vi "Flush Registry.vi"(8 "error in":errorcluster) -> (0 "error out":errorcluster)   [LabVIEW 2019, in "Identifier.lvclass"]
uses:
  Identifier.lvclass
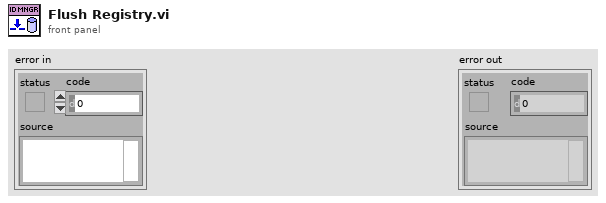
[diagram p1: front panel]
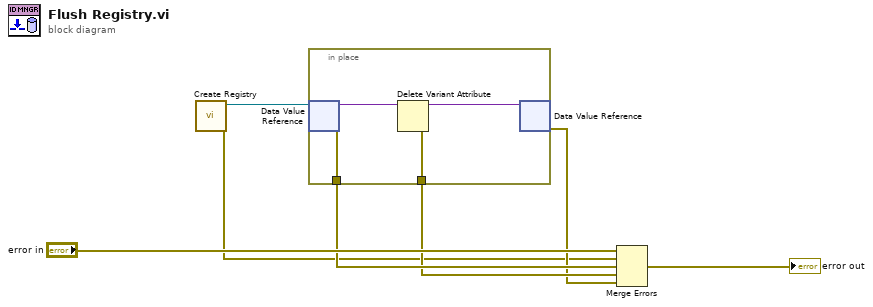
[diagram p0: block diagram]
diagram:
  n1 = call "Create Registry.vi"() -> ("error out"=w1:errorcluster, "Registry"=w6:refnum<data-value>)  [unwired: 10 in]
  n2 = in-place {
    in-place-border: [w9] -> w3
    in-place-border: [w8] -> w4
    n3 = in-place-dvr #1(w6) -> (w11:variant, w8:errorcluster)
    n4 = Delete Variant Attribute(7:w11) -> (0:w9:errorcluster, 3:w10:variant)  [unwired: 2 in, 1 out]
    n5 = in-place-dvr #1(w10) -> (w2:errorcluster)  [unwired: 1 out]
  }
  n6 = Merge Errors("error in", w1, w4, w3, w2) -> (→"error out":errorcluster)
